vi "ReadFromPTC10.vi"(8 "error in (no error)":errorcluster, 11 "PTC10":T1={"serial settings"={"port"="Stanford_PTC10", "baud rate"=9600}, "PTC10 Info"={"Manufacturer"="", "Instrument"="", "Serial Number"="", "Firmware"=""}, "VISA resource name"="", "pwmloop"="define pwmloop(#t=0 while (1) {waitforsample if(#pwm=0){relays=0}else{if(#t<#pwm) {relays=1}else{relays=3}}#t+=1 if  (#t>99){#t=0} pause 0.2 s})", "onecycle"="define onecycle (pwm=100 run pwmloop 5A.PID.Setpoint=-130.0 5A.PID.input=3C while(#3C>-129.0){pause 0.2 s}pwm=-130 pause 10 min pwm=0  5A.PID.SetPoint=50.0 while(#3C<49.0){pause 0.2 s} pause 10 min kill pwmloop)", "control"="define control (#count=1 while (#count>=0) {onecycle pause 1 s #count-=1})", "HeatDrive"="define Failsafe (while(1) {if (#Check <-20){relays=0 outputEnable Off}else{if(#Check>20){relays=0 outputEnable Off}} pause 1 s})", "ToAmbient"="define ToAmbient(if(#3C>25.0){pwm=100 run pwmloop while(#3C>#25.0){pause 0.5 s} pwm=0 kill pwmloop}else{#5A.PID.setpoint=20.0 while(#3C<15.0){pause 0.5 s} outputenable off})", "StartupCode"="system.display.Monitors Show", "LogChannels"=[], "Heater O/P Channel"="", " Control Input"="", "TAmbient"=20.0, "AmbientTolerance"=5.0, "PID Params"={"P"=1.14, "I"=0.012, "D"=21.68, "Set"=0.0}, "TestCycleParameters"={"TAmb"=20.0, "HeaterTestTemp"=20.0, "HeaterTestDwell(min)"=1, "HeaterTestDuration"=1, "MinOpTemp"=-131.5, "MinOpDwell(min)"=30, "TestHeatingRate (deg/min)"=0.4, "SurviveCycleParameters"={"MinSurviveTemp"=-131.5, "MinSurvive Dwell(min)"=10, "MaxSurviveTemp"=50.0, "MaxSurviveDwell(min)"=30, "ControlInput"=2, "ColdStandOff"=4.0, "HotStandoff"=5.0, "SteadyPWM"=20, "MaxCoolingRate (deg/min)"=3.75, "MaxHeatingRate (deg/min)"=2.5}, "CycleType"=0, "MaxOpTemp"=-50.0, "MaxOpDwell(min)"=30}} {"TestCycleParameters"."CycleType" items=["Survival", "Operational"]; "TestCycleParameters"."SurviveCycleParameters"."SteadyPWM" min=0 max=100 step=1; "TestCycleParameters"."SurviveCycleParameters"."ControlInput" items=["3A", "3B", "3C", "3D", "4A", "4B", "4C", "4D"]; "PID Params"."D" min=0.0; "PID Params"."I" min=0.0; "PID Params"."P" min=0.0; "TAmbient" min=0.0 max=30.0; "serial settings"."baud rate" items=["9600"=9600, "19200"=19200, "38400"=38400, "57600"=57600, "115200"=115200]}) -> (0 "error out":errorcluster, 1 "relays":i8=4, 2 "Cycles":i16, 3 "Temperature Chart":dynamicdata(graph), 4 "HeaterDrive":waveform(dbl)(graph), 5 "Target Temperature":dbl, 6 "Relay wfm":waveform(dbl))   [LabVIEW 2024]
uses:
  controls/SRS PTC10.ctl
  controls/PID Params.ctl
  controls/TestCycleParams.ctl
  controls/SurviveCycleParams.ctl
  controls/ControlInput.ctl
  <vilib>/Instr/_visa.llb/VISA Flush IO Buffer Mask.ctl
  Program Files/National Instruments/LabVIEW 2024/instr.lib/Stanford PTC10/SRS PTC10.lvlib
panel:
  in  "Tab Control":enum32{"Temperature", "Drive"}(tab)
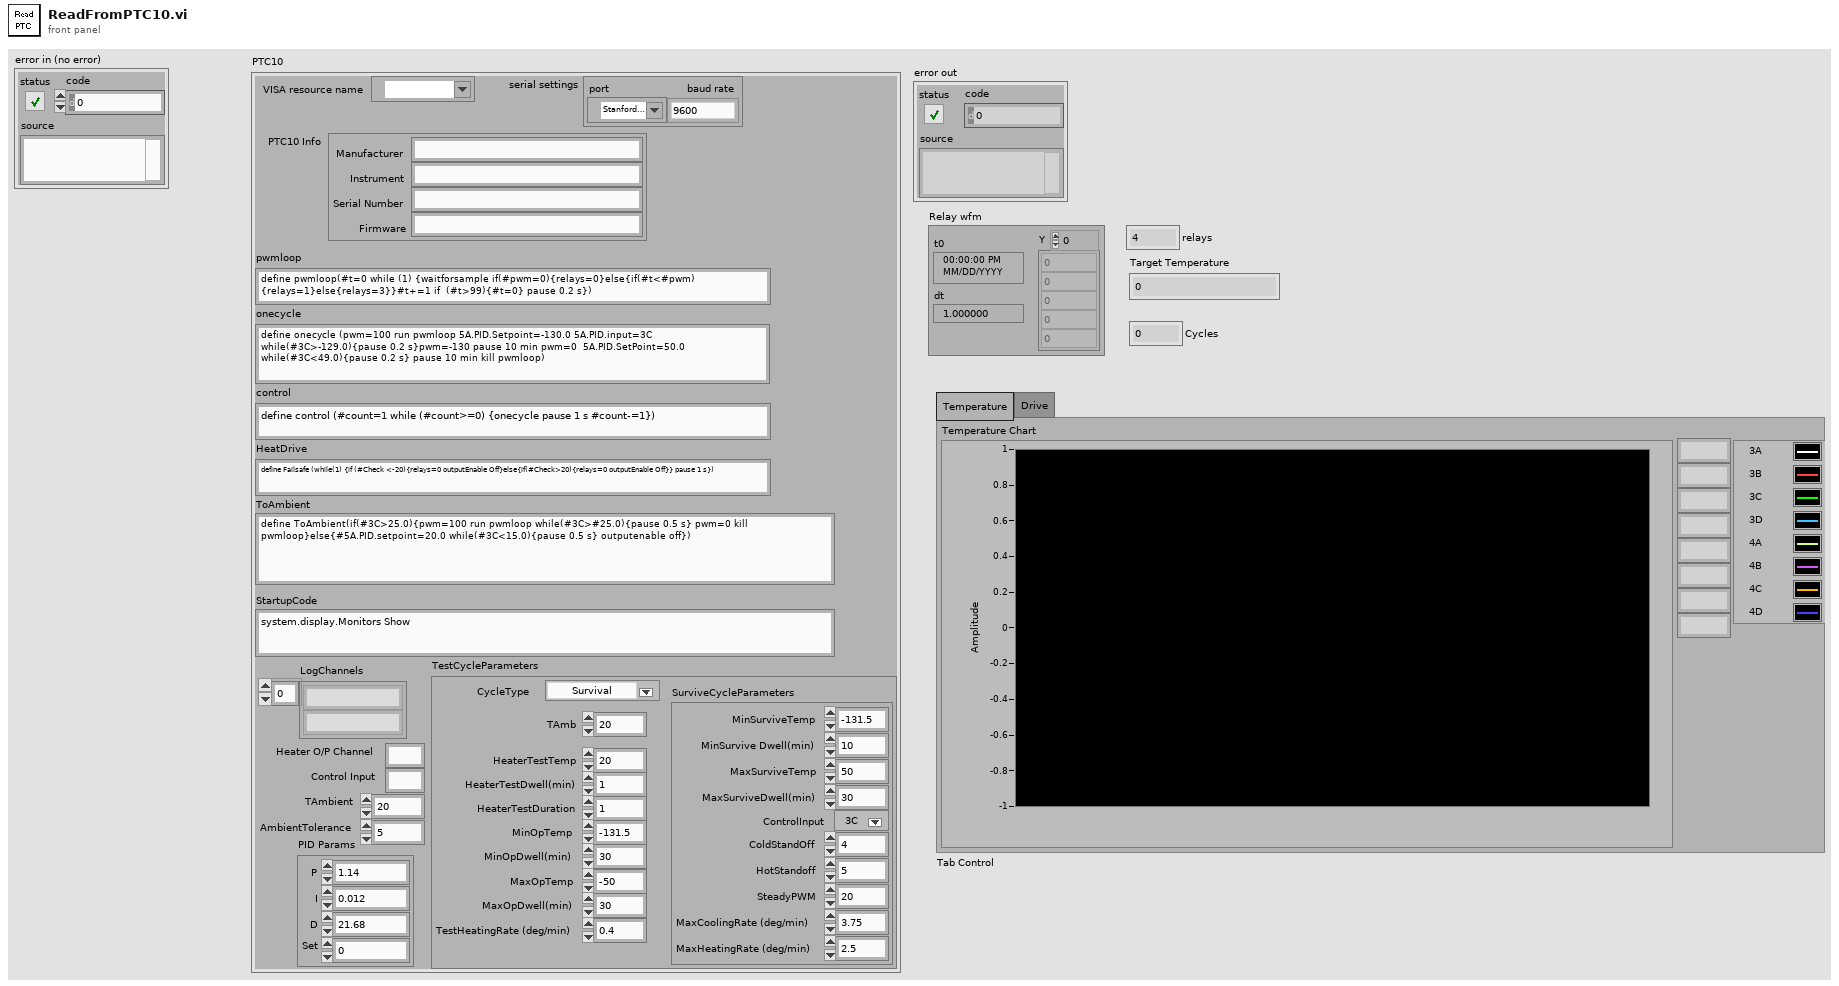
[diagram p1: front panel]
types:
  T1 = typedef "SRS PTC10.ctl" = cluster{"serial settings":cluster{"port":refnum<visa-resource-name>, "baud rate":u32}, "PTC10 Info":cluster{"Manufacturer":string, "Instrument":string, "Serial Number":string, "Firmware":string}, "VISA resource name":refnum<visa-resource-name>, "pwmloop":string, "onecycle":string, "control":string, "HeatDrive":string, "ToAmbient":string, "StartupCode":string, "LogChannels":string[], "Heater O/P Channel":string, " Control Input":string, "TAmbient":dbl, "AmbientTolerance":dbl, "PID Params":T2, "TestCycleParameters":T3}
  T2 = typedef "PID Params.ctl" = cluster{"P":dbl, "I":dbl, "D":dbl, "Set":dbl}
  T3 = typedef "TestCycleParams.ctl" = cluster{"TAmb":dbl, "HeaterTestTemp":dbl, "HeaterTestDwell(min)":i32, "HeaterTestDuration":i32, "MinOpTemp":dbl, "MinOpDwell(min)":i32, "TestHeatingRate (deg/min)":dbl, "SurviveCycleParameters":T4, "CycleType":u16, "MaxOpTemp":dbl, "MaxOpDwell(min)":i32}
  T4 = typedef "SurviveCycleParams.ctl" = cluster{"MinSurviveTemp":dbl, "MinSurvive Dwell(min)":i32, "MaxSurviveTemp":dbl, "MaxSurviveDwell(min)":i32, "ControlInput":T5, "ColdStandOff":dbl, "HotStandoff":dbl, "SteadyPWM":i32, "MaxCoolingRate (deg/min)":dbl, "MaxHeatingRate (deg/min)":dbl}
  T5 = typedef "ControlInput.ctl" = u16
  T6 = typedef "VISA Flush IO Buffer Mask.ctl" = u16
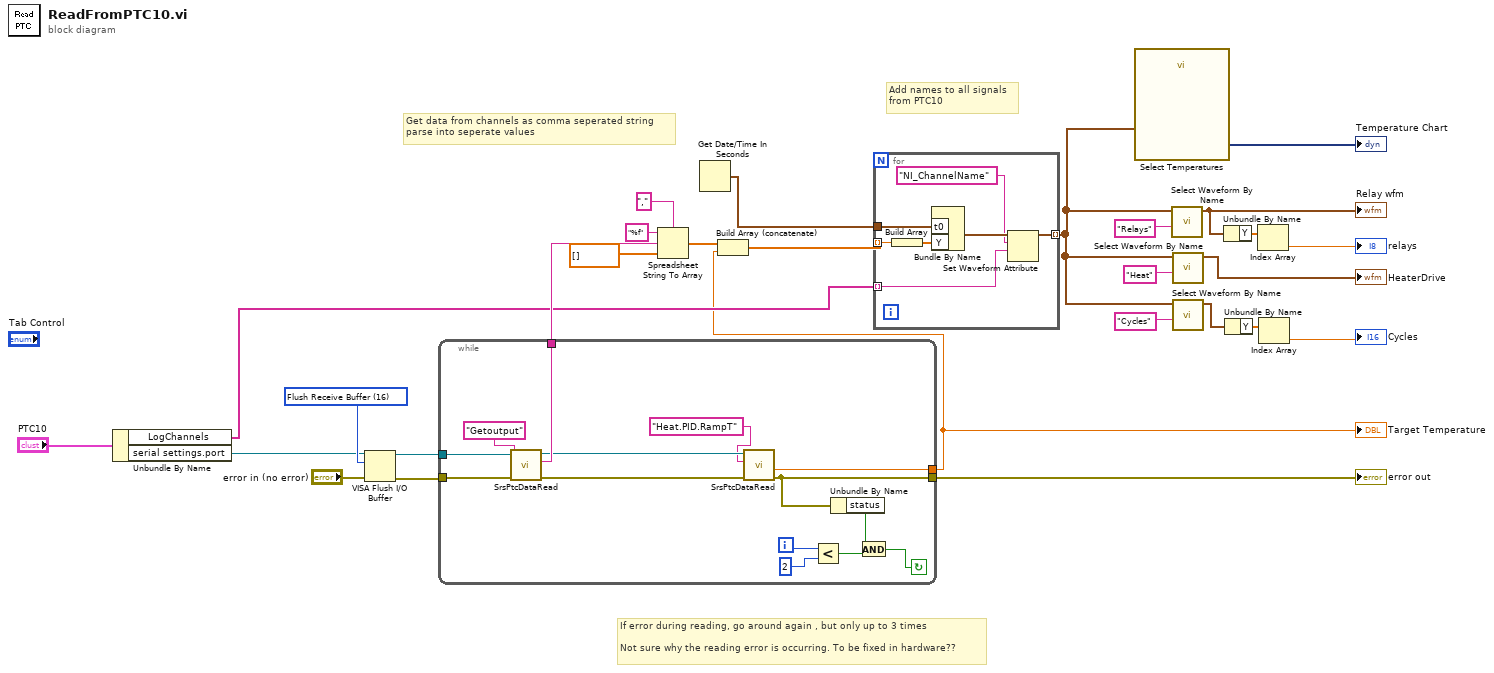
[diagram p0: block diagram]
diagram:
  w25 = T6 16 items=["Flush Receive Buffer"=16, "Write Transmit Buffer to Device"=32, "Flush Receive Buffer (No I/O)"=64, "Flush Transmit Buffer"=128] ("Mask")
  # "Get data from channels as comma seperated string\nparse into seperate values"
  # "Add names to all signals\nfrom PTC10"
  # "If error during reading, go around again , but only up to 3 times\n\nNot sure why the reading error is occurring. To be fixed in hardware??"
  n1 = Unbundle By Name("PTC10") -> ("LogChannels"=w17:string[], "serial settings.port"=w23:refnum<visa-resource-name>)
  n2 = VISA Flush I/O Buffer(VISA resource name=w23, mask (16)=w25, error in (no error)="error in (no error)") -> (VISA resource name out=w26:refnum<visa-resource-name>, error out=w27:errorcluster)
  n3 = while {
    tunnel: w26 -> [w41]
    tunnel: [w39] -> w22
    tunnel: [w35] -> w12
    tunnel: w27 -> [w42]
    tunnel: [w33] -> w16
    i -> [w30]
    stop <- w34 continue-if-true
    n4 = call "SrsPtcDataRead.vi"("error in"=w42, "Channel"="Getoutput", "SRS PTC10 VISA in"=w41) -> ("error out"=w38:errorcluster, "Output as text"=w39:string, "SRS PTC10 VISA out"=w37:refnum<visa-resource-name>)  [unwired: 5 in, 1 out]
    n5 = call "SrsPtcDataRead.vi"("error in"=w38, "Channel"="Heat.PID.RampT", "SRS PTC10 VISA in"=w37) -> ("error out"=w33:errorcluster, "Output as number"=w35:dbl)  [unwired: 5 in, 2 out]
    n6 = Less?(x=w30, y=2) -> (x < y?=w31:bool)
    n7 = Unbundle By Name(w33) -> ("status"=w32:bool)
    n8 = And(x=w32, y=w31) -> (x .and. y?=w34:bool)
  }
  "error out" <- w16
  "Target Temperature" <- w12
  n9 = Spreadsheet String To Array(delimiter (Tab)=",", format string="%f", spreadsheet string=w22, array type (2D Dbl)=dbl[] []) -> (array=w18:dbl[])
  n10 = Get Date/Time In Seconds() -> (seconds since 1Jan1904=w14:timestamp)
  n11 = Build Array (concatenate)(w18, w12) -> (w13:dbl[])
  n12 = for {
    tunnel: w13 -> [w48] mode=indexing
    tunnel: w17 -> [w45] mode=indexing
    tunnel: [w44] -> w2 mode=indexing
    tunnel: w14 -> [w43]
    n13 = Build Array(w48) -> (w47:dbl[])
    n14 = Bundle By Name("t0"=w43, "Y"=w47) -> (w49:waveform(dbl))  [unwired: 1 in]
    n15 = Set Waveform Attribute(5:w45, 6:"NI_ChannelName" ("name"), 7:w49) -> (3:w44:waveform(dbl))  [unwired: 1 in, 2 out]
  }
  n16 = call "Select Temperatures"("Signals"=w2) -> ("Signal Out"=→"Temperature Chart":dynamicdata)  [unwired: 9 in, 1 out]
  n17 = call "Select Waveform By Name.vi"("NI_ChannelName"="Relays" ("name"), "Array Of Wfm"=w2) -> ("Selected Wfm"=w8:waveform(dbl))  [unwired: 8 in, 1 out]
  "Relay wfm" <- w8
  n18 = call "Select Waveform By Name.vi"("NI_ChannelName"="Heat" ("name"), "Array Of Wfm"=w2) -> ("Selected Wfm"=→"HeaterDrive":waveform(dbl))  [unwired: 8 in, 1 out]
  n19 = call "Select Waveform By Name.vi"("NI_ChannelName"="Cycles" ("name"), "Array Of Wfm"=w2) -> ("Selected Wfm"=w3:waveform(dbl))  [unwired: 8 in, 1 out]
  n20 = Unbundle By Name(w8) -> ("Y"=w10:dbl[])
  n21 = Unbundle By Name(w3) -> ("Y"=w4:dbl[])
  n22 = Index Array(array=w10) -> (element=→"relays":dbl)  [unwired: 1 in]
  n23 = Index Array(array=w4) -> (element=→"Cycles":dbl)  [unwired: 1 in]
